vi "设置窗口.vi"() -> (3 "确定输出":bool)   [LabVIEW 2016, in "ADCP.lvlib"]
uses:
  ADCP.lvlib
panel:
  in  "层数":u16=1 caption="层          数" min=1 max=128 step=1
  in  "ADCP类型":string(combo)="在线ADCP"
  in  "ADCP型号":string(combo)
  in  "串口":refnum<visa-resource-name>="COM6"
  in  "串口开关":bool
  in  "取消":bool
  in  "确定":bool
  # "设置ADCP参数"
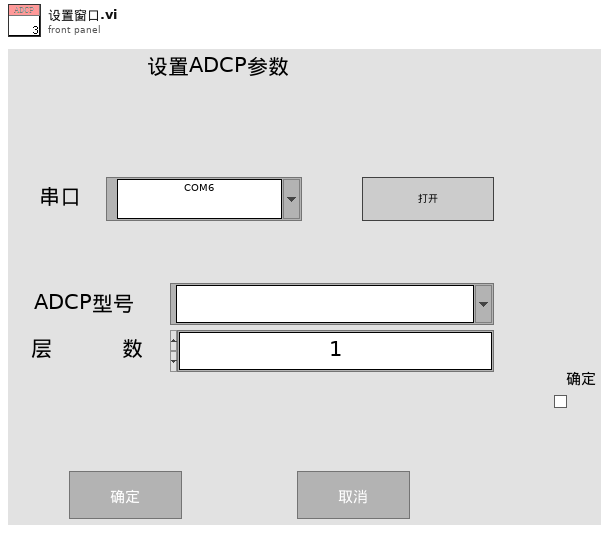
[diagram p1: front panel]
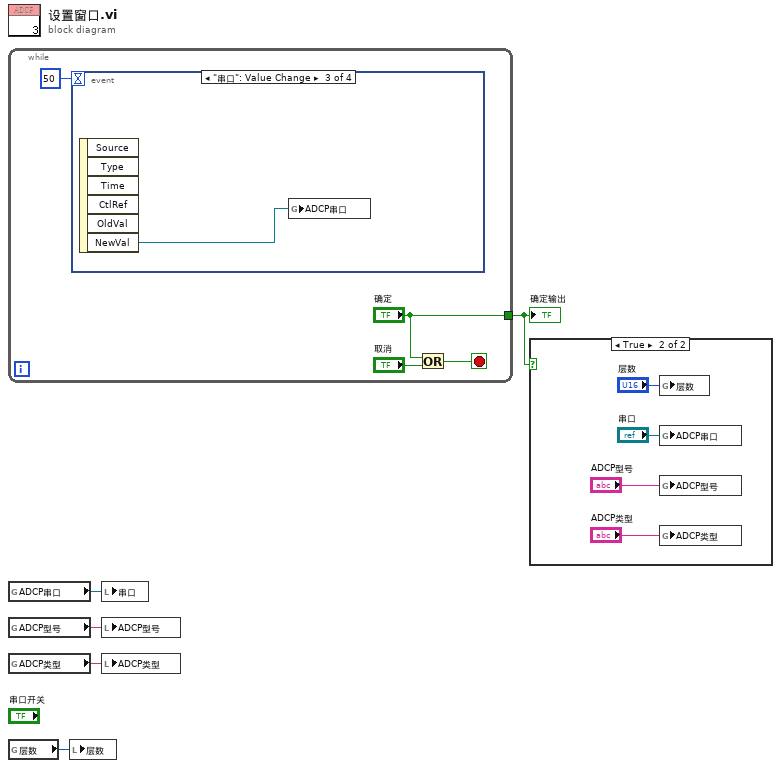
[diagram p0: block diagram]
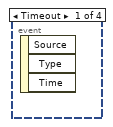
[diagram p3: hidden frame]
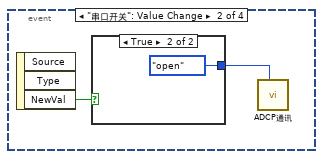
[diagram p4: hidden frame]
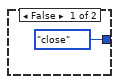
[diagram p5: hidden frame]
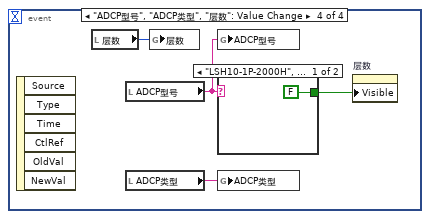
[diagram p6: hidden frame]
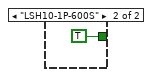
[diagram p7: hidden frame]
diagram:
  n1 = while {
    tunnel: ["确定"] -> w5
    stop <- w8 stop-if-true
    n2 = event shown="[2] \"串口\": Value Change" {
      selector: _ -> [_ _ _ _]
      dyn-events: _ -> [_ _ _ _]
      timeout: 50 -> [_ _ _ _]
      event Timeout {
        n3 = event-data() -> ()  [unwired: 1 in, 3 out]
      }
      event "串口开关": Value Change {
        n4 = event-data() -> ("NewVal"=w10:bool)  [unwired: 1 in, 2 out]
        n5 = case shown="True" w10 {
          tunnel: [enum16{"open", "read", "write", "close"}."close" ("STEP") enum16{"open", "read", "write", "close"}."open" ("STEP")] -> w11
          frame False {
          }
          frame True {
          }
        }
        n6 = call "ADCP通讯.vi"("STEP"=w11) -> ()  [unwired: 8 in, 3 out]
      }
      event "串口": Value Change {
        n7 = event-data() -> ("NewVal"=w14:refnum<visa-resource-name>)  [unwired: 1 in, 5 out]
        n8 = global write "ADCP全局变量.vi" "ADCP串口"(w14) -> ()
      }
      event "ADCP型号", "ADCP类型", "层数": Value Change {
        n9 = event-data() -> ()  [unwired: 1 in, 6 out]
        n10 = local read "层数"() -> (w17:u16)
        n11 = local read "ADCP型号"() -> (w16:string)
        n12 = local read "ADCP类型"() -> (w18:string)
        n13 = global write "ADCP全局变量.vi" "层数"(w17) -> ()
        n14 = global write "ADCP全局变量.vi" "ADCP型号"(w16) -> ()
        n15 = case shown="\"LSH10-1P-2000H\", Default" w16 {
          tunnel: [FALSE TRUE] -> w15
          frame "LSH10-1P-2000H", Default {
          }
          frame "LSH10-1P-600S" {
          }
        }
        n16 = global write "ADCP全局变量.vi" "ADCP类型"(w18) -> ()
        n17 = property on="层数" class="DigNum (strict)"("Visible"=w15) -> ()  [unwired: 2 in, 2 out]
      }
    }
    n18 = Or(x="确定", y="取消") -> (x .or. y?=w8:bool)
  }
  "确定输出" <- w5
  n19 = global read "ADCP全局变量.vi" "ADCP串口"() -> (w4:refnum<visa-resource-name>)
  n20 = global read "ADCP全局变量.vi" "ADCP型号"() -> (w3:string)
  n21 = global read "ADCP全局变量.vi" "ADCP类型"() -> (w2:string)
  n22 = global read "ADCP全局变量.vi" "层数"() -> (w1:u16)
  n23 = local write "层数"(w1) -> ()
  n24 = local write "串口"(w4) -> ()
  n25 = local write "ADCP型号"(w3) -> ()
  n26 = local write "ADCP类型"(w2) -> ()
  n27 = case shown="True" w5 {
    frame False {
    }
    frame True {
      n28 = global write "ADCP全局变量.vi" "层数"("层数") -> ()
      n29 = global write "ADCP全局变量.vi" "ADCP串口"("串口") -> ()
      n30 = global write "ADCP全局变量.vi" "ADCP型号"("ADCP型号") -> ()
      n31 = global write "ADCP全局变量.vi" "ADCP类型"("ADCP类型") -> ()
    }
  }
